vi "ui_close_connection.vi"(8 "error in (no error)":errorcluster caption="错误输入（无错误）") -> (0 "error out":errorcluster caption="错误输出")   [LabVIEW 2015]
uses:
  globals/global_ui_stream_and_variable_connections.vi
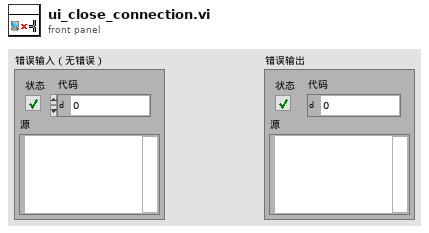
[diagram p1: front panel]
types:
  T1 = typedef "variable_references.ctl" = cluster{"CPU 1 Usage":refnum<k21>, "Free Memory":refnum<k21>, "Actual Loop Period":refnum<k21>, "CPU 2 Usage":refnum<k21>, "Drive Space":refnum<k21>, "Number of Data Files":refnum<k21>, "System Time":refnum<k21>}
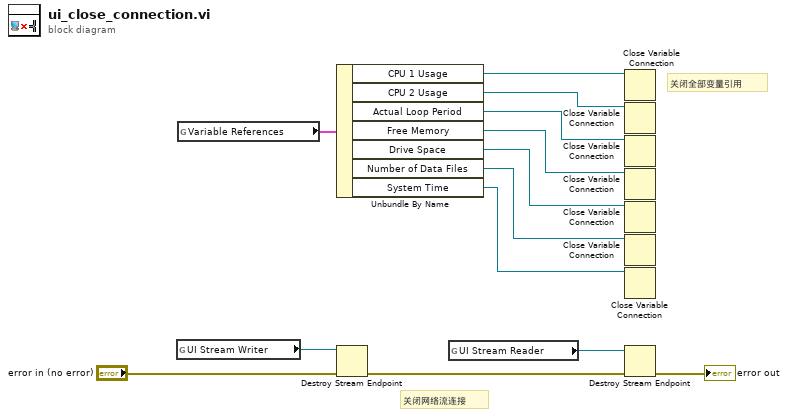
[diagram p0: block diagram]
diagram:
  # "关闭网络流连接"
  # "关闭全部变量引用"
  n1 = global read "global_ui_stream_and_variable_connections.vi" "UI Stream Writer"() -> (w3:refnum<k21>)
  n2 = global read "global_ui_stream_and_variable_connections.vi" "Variable References"() -> (w6:T1)
  n3 = Unbundle By Name(w6) -> ("CPU 1 Usage"=w10:refnum<k21>, "CPU 2 Usage"=w11:refnum<k21>, "Actual Loop Period"=w12:refnum<k21>, "Free Memory"=w13:refnum<k21>, "Drive Space"=w9:refnum<k21>, "Number of Data Files"=w8:refnum<k21>, "System Time"=w7:refnum<k21>)
  n4 = Destroy Stream Endpoint(8:"error in (no error)", 11:w3) -> (0:w4:errorcluster)
  n5 = global read "global_ui_stream_and_variable_connections.vi" "UI Stream Reader"() -> (w5:refnum<k21>)
  n6 = Close Variable Connection(11:w10) -> ()  [unwired: 1 in, 1 out]
  n7 = Close Variable Connection(11:w11) -> ()  [unwired: 1 in, 1 out]
  n8 = Close Variable Connection(11:w12) -> ()  [unwired: 1 in, 1 out]
  n9 = Close Variable Connection(11:w13) -> ()  [unwired: 1 in, 1 out]
  n10 = Close Variable Connection(11:w9) -> ()  [unwired: 1 in, 1 out]
  n11 = Close Variable Connection(11:w8) -> ()  [unwired: 1 in, 1 out]
  n12 = Close Variable Connection(11:w7) -> ()  [unwired: 1 in, 1 out]
  n13 = Destroy Stream Endpoint(8:w4, 11:w5) -> (0:→"error out":errorcluster)
